vi "Decorator.vi"(6 "Sender":refnum<class "Sender.lvclass">, 7 "Actor in":refnum<class "Actor.lvclass">) -> (0 "Error out":errorcluster, 5 "Actor out":refnum<class "Actor.lvclass">)   [LabVIEW 2025, in "_Template.lvlib" / "Templates.lvlib" / "TEMPLATE Msg.lvlib"]
uses:
  TEMPLATE Msg.lvlib
  jettl/jettl/Actor/Actor/Actor.lvclass
  jettl/jettl/Sender/Sender/Sender.lvclass
  TEMPLATE Msg/TEMPLATE Msg.lvclass
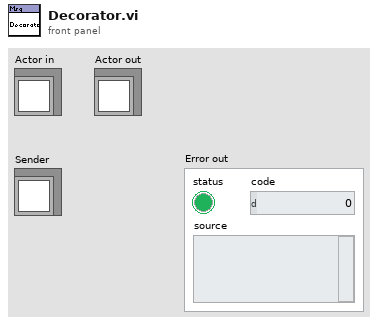
[diagram p1: front panel]
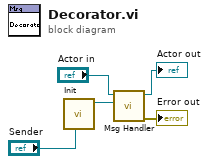
[diagram p0: block diagram]
diagram:
  n1 = call "Init.vi"("Sender"="Sender") -> ("TEMPLATE Msg out"=w2:refnum<class "TEMPLATE Msg.lvclass">)  [unwired: 10 in]
  n2 = call-dynamic "Msg Handler.vi"("Msg"=w2, "Actor in"="Actor in") -> ("Error out"=→"Error out":errorcluster, "Actor out"=→"Actor out":refnum<class "Actor.lvclass">)  [unwired: 8 in]
